vi "lab2RectangleArea.vi"(1 "Rectangle":T1) -> (0 "Area":u32)   [LabVIEW 2016]
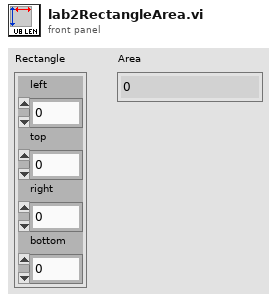
[diagram p1: front panel]
types:
  T1 = cluster{"left":i16, "top":i16, "right":i16, "bottom":i16}
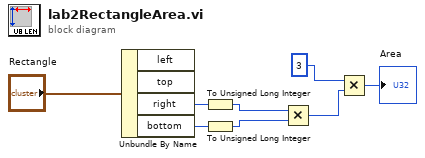
[diagram p0: block diagram]
diagram:
  n1 = Unbundle By Name("Rectangle") -> ("right"=w6:i16, "bottom"=w7:i16)  [unwired: 2 out]
  n2 = To Unsigned Long Integer(number=w6) -> (unsigned 32bit integer=w5:u32)
  n3 = To Unsigned Long Integer(number=w7) -> (unsigned 32bit integer=w4:u32)
  n4 = Multiply(x=w5, y=w4) -> (x*y=w2:u32)
  n5 = Multiply(x=u32 3, y=w2) -> (x*y=→"Area":u32)
